vi "Monitor Homed Status.vi"(8 "error in (no error)":errorcluster, 9 "Y-Axis In":refnum<class "iMotion Controller.lvclass">, 10 "X-Axis In":refnum<class "iMotion Controller.lvclass">, 11 "Stage Data Class":refnum<data-value>) -> (0 "error out":errorcluster, 1 "Y-Axis Out":refnum<class "iMotion Controller.lvclass">, 2 "X-Axis Out":refnum<class "iMotion Controller.lvclass">, 3 "Stage Data Class":refnum<data-value>)   [LabVIEW 2022 SP3, in "XY Stage Process.lvlib" / "XY Stage Process.lvclass"]
uses:
  XY Stage Process.lvclass
  XY Stage Process.lvclass/XY Stage Process.ctl
  Axis Objects/iMotion Controller/iMotion Controller.lvclass
  XY Stage Data Class/Homed.ctl
  XY Stage Data Class/XY Stage Data Class.lvclass
  6046c730-44da-4461-abcf-74f1f8a9aa6a.vi
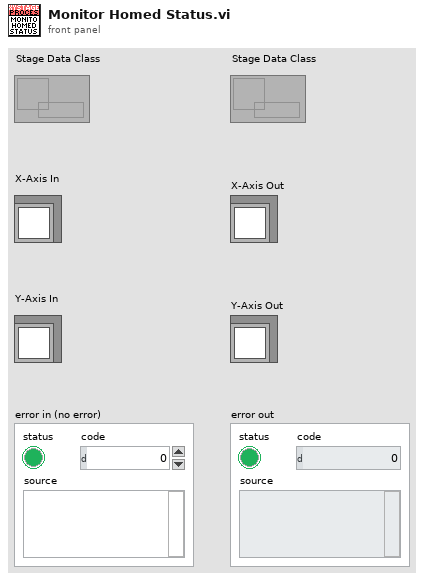
[diagram p1: front panel]
types:
  T1 = typedef "XY Stage Data Class.lvclass/Homed.ctl" = cluster{"X Homed":bool, "Y Homed":bool}
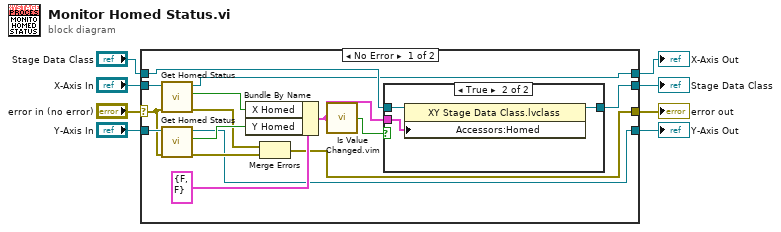
[diagram p0: block diagram]
diagram:
  n1 = case shown="No Error" "error in (no error)" {
    selector: "error in (no error)" -> [w15 w28]
    tunnel: "Y-Axis In" -> [w18 w29]
    tunnel: "X-Axis In" -> [w17 w30]
    tunnel: "Stage Data Class" -> [w16 w31]
    tunnel: [w12 w31] -> w4
    tunnel: [w11 w30] -> w3
    tunnel: [w10 w29] -> w2
    tunnel: [w9 w28] -> w1
    frame No Error {
      n2 = call-dynamic "Get Homed Status.vi"("error in (no error)"=w15, "iMotion Controller in"=w17) -> ("error out"=w14:errorcluster, "Homed"=w19:bool, "iMotion Controller out"=w11:refnum<class "iMotion Controller.lvclass">)  [unwired: 7 in]
      n3 = call-dynamic "Get Homed Status.vi"("error in (no error)"=w15, "iMotion Controller in"=w18) -> ("error out"=w13:errorcluster, "Homed"=w21:bool, "iMotion Controller out"=w10:refnum<class "iMotion Controller.lvclass">)  [unwired: 7 in]
      n4 = Bundle By Name(cluster=T1 {"X Homed"=FALSE, "Y Homed"=FALSE} ("Homed"), "X Homed"=w19, "Y Homed"=w21) -> (w22:T1)
      n5 = Merge Errors(w14, w13) -> (w9:errorcluster)
      n6 = call "Is Value Changed.vim"("value"=w22) -> ("changed or first call?"=w23:bool)
      n7 = case shown="True" w23 {
        tunnel: w22 -> [_ w25]
        tunnel: [w24 w27] -> w12
        tunnel: w16 -> [w24 w26]
        frame False {
        }
        frame True {
          n8 = property class="XY Stage Data Class.lvclass"(reference=w26, "Accessors:Homed"=w25) -> (reference out=w27:refnum<data-value>)  [unwired: 1 in, 1 out]
        }
      }
    }
    frame Error {
    }
  }
  "Stage Data Class" <- w4
  "X-Axis Out" <- w3
  "Y-Axis Out" <- w2
  "error out" <- w1
